vi "Indice registri.vi"(10 "Lista tipi di parametro":T1=14 items=["Table of parameters (P00-P199)", "Table of connections (C00-C99)", "Table of application parameters (E00-E99)", "Table of expanded application parameters (E100-E600)", "Table of internal values (D00-D127)", "Drive state", "Drive alarms", "Alarm enabling", "Speed reference from fieldbus", "Torque limit from fieldbus", "Torque reference from fieldbus", "Mechanical position read", "Logic functions of digital input", "Logic funtction of digital input from serial c.", "logical function of standard digital outputs", "logic function of application digital output", "Table of parameters formats", "Table of connections formats", "Table of monitor and analog outputs values", "Table of application parameters formats", "Table of internal values formats"], 11 "Mappa registri":string[][](array[string])) -> (1 "Array registri":i32[](array[numeric]), 2 "Numero registri":i32, 3 "Registro iniziale":i32)   [LabVIEW 2019]
uses:
  Tipi di parametro.ctl
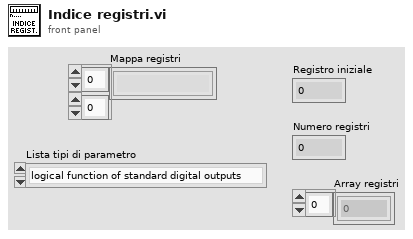
[diagram p1: front panel]
types:
  T1 = typedef "Tipi di parametro.ctl" = u16
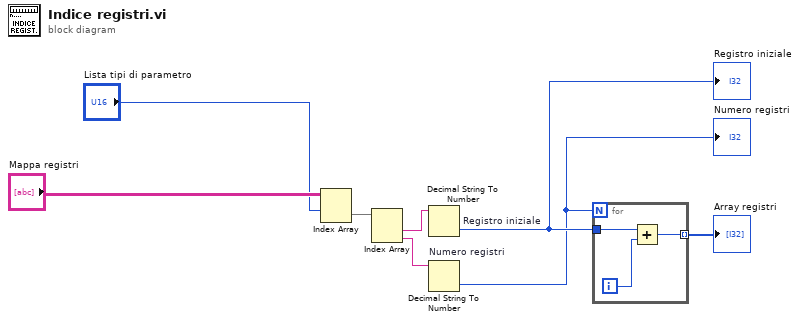
[diagram p0: block diagram]
diagram:
  n1 = Index Array(array="Mappa registri", index (row)="Lista tipi di parametro") -> (element=w2:string[])  [unwired: 1 in]
  n2 = Index Array(array=w2) -> (element #1=w3:string, element #2=w4:string)  [unwired: 2 in]
  n3 = Decimal String To Number "Registro iniziale"(string=w3) -> (number=w6:i32)  [unwired: 2 in, 1 out]
  "Registro iniziale" <- w6
  n4 = Decimal String To Number "Numero registri"(string=w4) -> (number=w5:i32)  [unwired: 2 in, 1 out]
  "Numero registri" <- w5
  n5 = for {
    N: w5 -> [_]
    tunnel: w6 -> [w11]
    tunnel: [w9] -> w7 mode=indexing
    i -> [w10]
    n6 = Add(x=w11, y=w10) -> (x+y=w9:i32)
  }
  "Array registri" <- w7
